vi "Generate_events.vi"(8 "error in (no error)":errorcluster, 10 "Game in":refnum<class "Game.lvclass">, 11 "Events in":refnum<class "Events.lvclass">) -> (0 "error out":errorcluster, 1 "kick":bool, 2 "touch":bool, 3 "Events out":refnum<class "Events.lvclass">)   [LabVIEW 2023, in "Events.lvclass"]
uses:
  Events.lvclass
  Events.lvclass/Events.ctl
  Game_class/Game.lvclass
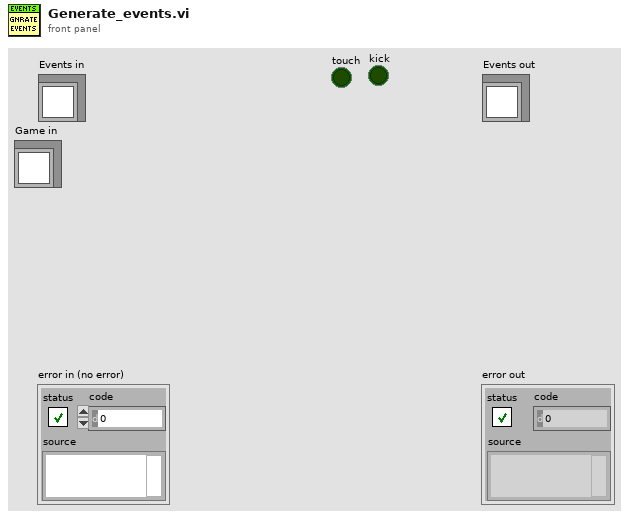
[diagram p1: front panel]
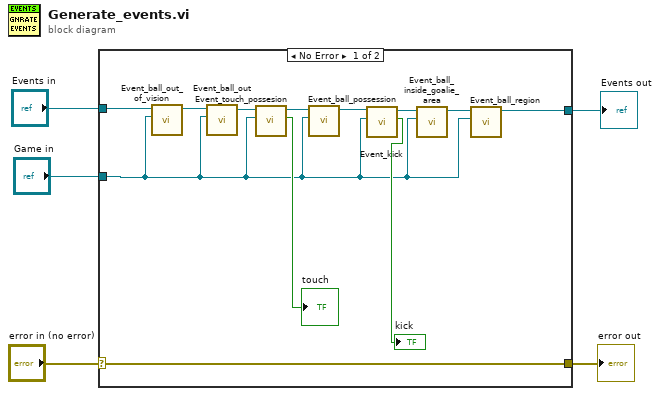
[diagram p0: block diagram]
diagram:
  n1 = case shown="No Error" "error in (no error)" {
    selector: "error in (no error)" -> [w17 w19]
    tunnel: [w17 w19] -> w4
    tunnel: [w12 w18] -> w2
    tunnel: "Events in" -> [w16 w18]
    tunnel: "Game in" -> [w6 _]
    frame No Error {
      n2 = call-dynamic "Event_ball_out_of_vision.vi"("Game in"=w6, "Events in"=w16) -> ("Events out"=w15:refnum<class "Events.lvclass">)  [unwired: 8 in, 1 out]
      n3 = call "Event_ball_out.vi"("Game in"=w6, "Events in"=w15) -> ("Events out"=w11:refnum<class "Events.lvclass">)  [unwired: 8 in, 1 out]
      n4 = call-dynamic "Event_touch_possesion.vi"("Game in"=w6, "Events in"=w11) -> ("touch"=→"touch":bool, "Events out"=w10:refnum<class "Events.lvclass">)  [unwired: 7 in, 1 out]
      n5 = call-dynamic "Event_ball_possession.vi"("Game"=w6, "Events in"=w10) -> ("Events out"=w9:refnum<class "Events.lvclass">)  [unwired: 8 in, 1 out]
      n6 = call-dynamic "Event_kick.vi"("Game"=w6, "Events in"=w9) -> ("kick"=→"kick":bool, "Events out"=w14:refnum<class "Events.lvclass">)  [unwired: 7 in, 1 out]
      n7 = call "Event_ball_inside_goalie_area.vi"("Game in"=w6, "Events in"=w14) -> ("Events out"=w7:refnum<class "Events.lvclass">)  [unwired: 8 in, 1 out]
      n8 = call-dynamic "Event_ball_region.vi"("Game in"=w6, "Events in"=w7) -> ("Events out"=w12:refnum<class "Events.lvclass">)  [unwired: 8 in, 1 out]
    }
    frame Error {
    }
  }
  "error out" <- w4
  "Events out" <- w2
